vi "MGI RWA Anything to String.vi"(8 "Error In":errorcluster, 9 "Anything":variant, 10 "Read/Write Options":T1={"TS Fmt"="", "Int Fmt"="", "Delimiter"=","}, 11 "Format String (%#_13g)":string="%#_13g") -> (0 "Error Out":errorcluster, 1 "Section":string, 2 "Strings[]":string[](array[string]), 4 "Warnings":string)   [LabVIEW 2023]
doc: "Output a string representation of the specified datatype.\n\nAuthored by Robert C. Mortensen\nsupport@mooregoodideas.com\nwww.mooregoodideas.com\n\nCopyright (c) 2010, Moore Good Ideas, Inc.\n\nAll rights reserved.\n\nRedistribution and use in source and binary forms, with or without modification, are permitted provided that the following conditions are met:\n\n * Redistributions of source code must retain the above copyright notice, this list of conditions and the following disclaimer.\n * Redistributions in binary form must reproduce the above copyright notice, this list of conditions and the following disclaimer in the documentation and/or other materials provided with the distribution.\n * Neither the name of Moore Good Ideas, Inc. nor the names of its contributors may be used to endorse or promote products derived from this software without specific prior written permission.\n\nTHIS SOFTWARE IS PROVIDED BY THE COPYRIGHT HOLDERS AND CONTRIBUTORS \"AS IS\" AND ANY EXPRESS OR IMPLIED WARRANTIES, INCLUDING, BUT NOT LIMITED TO, THE IMPLIED WARRANTIES OF MERCHANTABILITY AND FITNESS FOR A PARTICULAR PURPOSE ARE DISCLAIMED. IN NO EVENT SHALL THE COPYRIGHT OWNER OR CONTRIBUTORS BE LIABLE FOR ANY DIRECT, INDIRECT, INCIDENTAL, SPECIAL, EXEMPLARY, OR CONSEQUENTIAL DAMAGES (INCLUDING, BUT NOT LIMITED TO, PROCUREMENT OF SUBSTITUTE GOODS OR SERVICES; LOSS OF USE, DATA, OR PROFITS; OR BUSINESS INTERRUPTION) HOWEVER CAUSED AND ON ANY THEORY OF LIABILITY, WHETHER IN CONTRACT, STRICT LIABILITY, OR TORT (INCLUDING NEGLIGENCE OR OTHERWISE) ARISING IN ANY WAY OUT OF THE USE OF THIS SOFTWARE, EVEN IF ADVISED OF THE POSSIBILITY OF SUCH DAMAGE."
uses:
  MGI RWA Options Cluster.ctl
  MGI RWA Convertion Direction Enum.ctl
  <vilib>/Utility/Data Type/NI_Data Type.lvlib
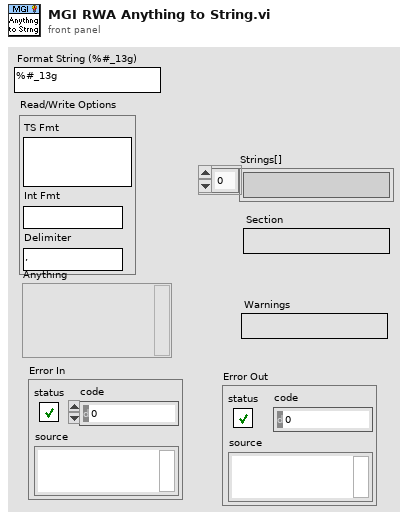
[diagram p1: front panel]
types:
  T1 = typedef "MGI RWA Options Cluster.ctl" = cluster{"TS Fmt":string, "Int Fmt":string, "Delimiter":string}
  T2 = typedef "MGI RWA Convertion Direction Enum.ctl" = enum16{"String->Anything", "Anything->String"}
  T3 = typedef "MGI RWA Tag Lookup Cluster.ctl" = cluster{"StrToSpecifiedText":variant, "Specified Data":variant, "Float Fmt":string, "Major Vers":i32, "Options":T1}
  T4 = typedef "NI_Data Type.lvlib/Data Type.ctl" = enum8{"Invalid Type", "Void", "I8", "I16", "I32", "I64", "U8", "U16", "U32", "U64", "Single Float", "Double Float", "Extended Float", "Single Complex", "Double Complex", "Extended Complex", "Enum U8", "Enum U16", "Enum U32", "Enum U64", "Single Float With Unit", "Double Float With Unit", "Extended Float With Unit", "Single Complex with Unit", "Double Complex with Unit", "Extended Complex with Unit", "Boolean", "String", "Path", "Picture", "Tag", "Array", "Cluster", "Variant", "LV Variant", "Waveform", "Timestamp", "Digital Waveform", "Digital Data", "ExpressData", "Refnum", "External Data", "VI", "Poly VI", "LabVIEW Class Instance", "Fixed Point", "Set Collection", "Map Collection"}
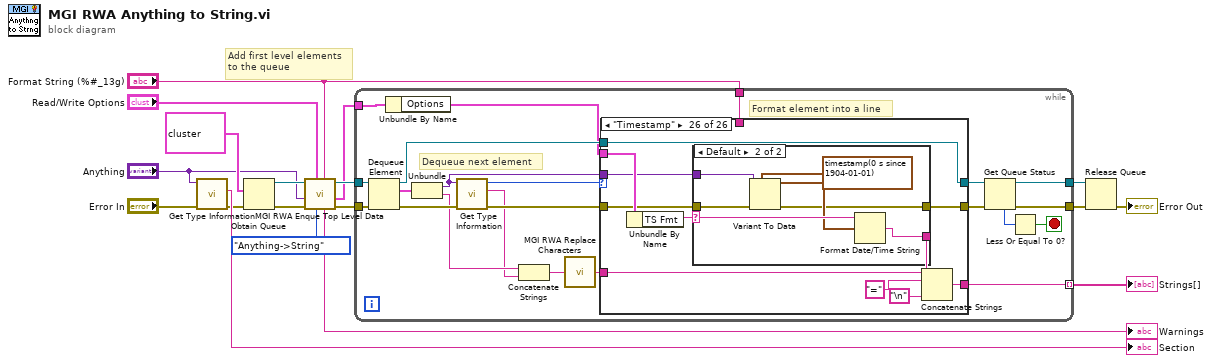
[diagram p0: block diagram]
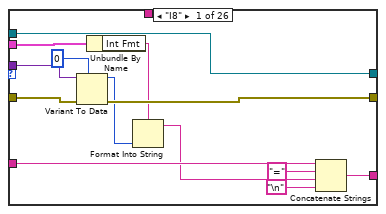
[diagram p2: hidden frame]
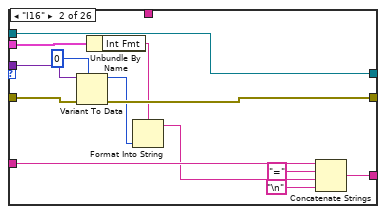
[diagram p3: hidden frame]
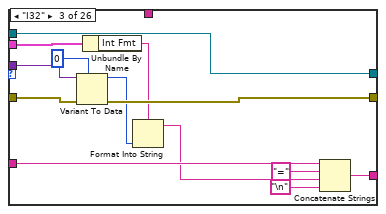
[diagram p4: hidden frame]
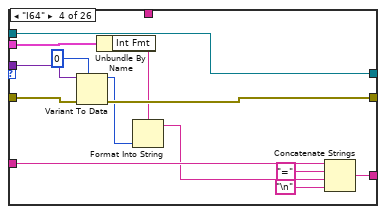
[diagram p5: hidden frame]
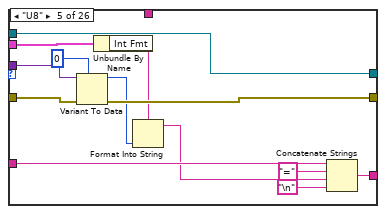
[diagram p6: hidden frame]
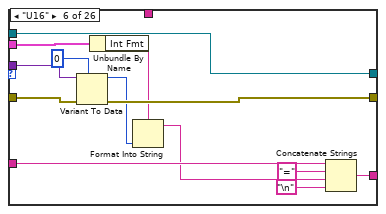
[diagram p7: hidden frame]
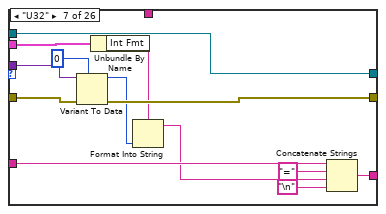
[diagram p8: hidden frame]
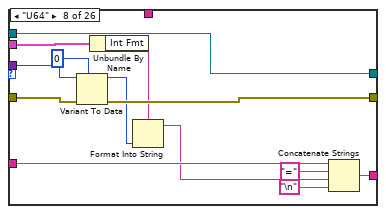
[diagram p9: hidden frame]
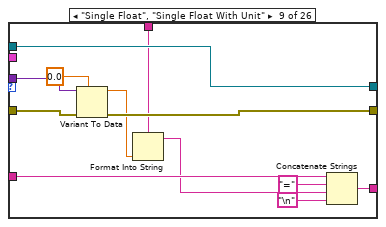
[diagram p10: hidden frame]
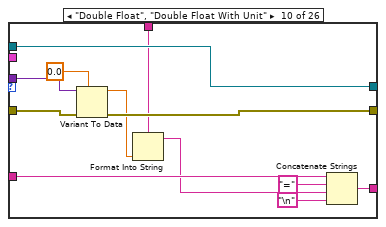
[diagram p11: hidden frame]
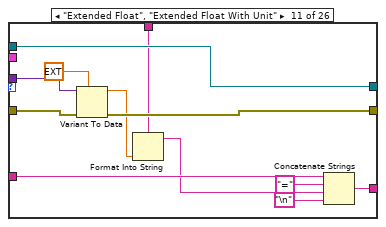
[diagram p12: hidden frame]
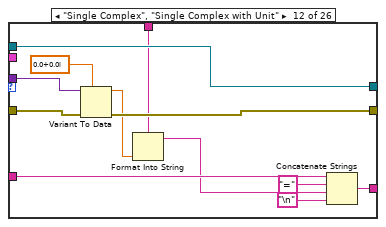
[diagram p13: hidden frame]
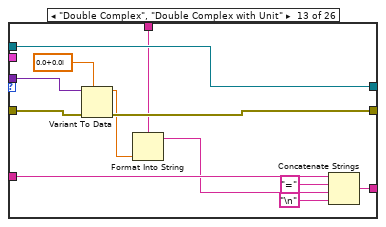
[diagram p14: hidden frame]
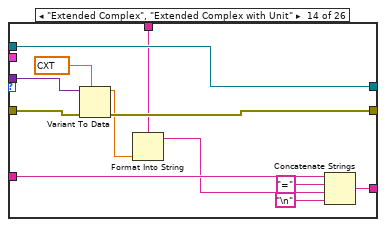
[diagram p15: hidden frame]
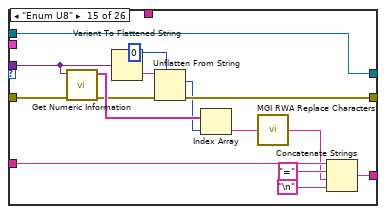
[diagram p16: hidden frame]
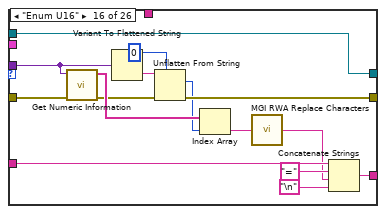
[diagram p17: hidden frame]
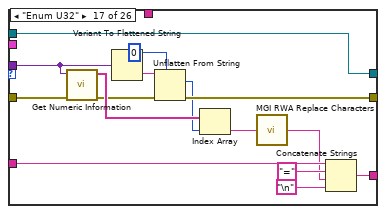
[diagram p18: hidden frame]
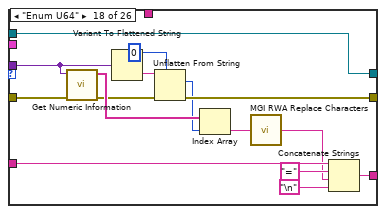
[diagram p19: hidden frame]
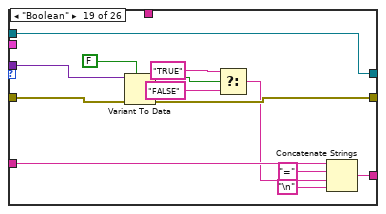
[diagram p20: hidden frame]
diagram:
  # "Add first level elements\nto the queue"
  n1 = call <vilib>:"Get Type Information.vi"("error in (no error)"="Error In", "variant"="Anything") -> ("error out"=w4:errorcluster, "name"=→"Section":string)  [unwired: 5 in, 3 out]
  n2 = Obtain Queue(element data type=cluster{"Variant":variant, "Name":string} {"Variant"=variant, "Name"=""}, error in (no error)=w4) -> (queue out=w10:refnum<queue>, error out=w11:errorcluster)  [unwired: 3 in, 1 out]
  n3 = call "MGI RWA Enque Top Level Data.vi"("Format String (%#_13g)"="Format String (%#_13g)", "Conversion"=MGI_RWA_Convertion_Direction_Enum."Anything->String", "Read/Write Options"="Read/Write Options", "Error In"=w11, "Anything"="Anything", "Data Queue In"=w10) -> ("Error Out"=w6:errorcluster, "Read State"=w2:T3, "Data Queue Our"=w5:refnum<queue>, "Warnings"=→"Warnings":string)  [unwired: 1 in, 1 out]
  n4 = while {
    tunnel: w6 -> [w40]
    tunnel: [w37] -> w12
    tunnel: [w25] -> w18 mode=indexing
    tunnel: w5 -> [w38]
    tunnel: [w34] -> w13
    tunnel: "Format String (%#_13g)" -> [w21]
    tunnel: w2 -> [w20]
    stop <- w35 stop-if-true
    # "Format element into a line"
    # "Dequeue next element"
    n5 = Dequeue Element(queue=w38, error in (no error)=w40) -> (queue out=w31:refnum<queue>, element=w29:cluster{"Variant":variant, "Name":string}, error out=w39:errorcluster)  [unwired: 1 in, 1 out]
    n6 = Unbundle By Name(w20) -> ("Options"=w19:T1)
    n7 = Unbundle(w29) -> ("Variant"=w28:variant, "Name"=w27:string)
    n8 = call <vilib>:"Get Type Information.vi"("error in (no error)"=w39, "variant"=w28) -> ("error out"=w26:errorcluster, "name"=w24:string, "type"=w33:T4)  [unwired: 5 in, 2 out]
    n9 = Concatenate Strings(w27, w24) -> (w23:string)
    n10 = call "MGI RWA Replace Characters.vi"("String In"=w23) -> ("String Out"=w22:string)  [unwired: 1 in]
    n11 = case shown="\"Timestamp\"" w33 {
      selector: w33 -> [_ _ _ _ _ _ _ _ _ _ _ _ _ _ _ _ _ _ _ _ _ _ w330 _ _ _]
      tunnel: [w53 w66 w79 w92 w105 w118 w131 w144 w156 w168 w180 w192 w204 w216 w231 w246 w261 w276 w289 w300 w312 w320 w334 w356 w364 w374] -> w32
      tunnel: w31 -> [w53 w66 w79 w92 w105 w118 w131 w144 w156 w168 w180 w192 w204 w216 w231 w246 w261 w276 w289 w300 w312 w324 w335 w356 w364 w374]
      tunnel: [w49 w62 w75 w88 w101 w114 w127 w140 w152 w164 w176 w188 w200 w212 w225 w240 w255 w270 w288 w292 w311 w321 w336 w355 w363 w367] -> w30
      tunnel: w26 -> [w52 w65 w78 w91 w104 w117 w130 w143 w155 w167 w179 w191 w203 w215 w230 w245 w260 w275 w285 w295 w308 w322 w332 w355 w365 w368]
      tunnel: w22 -> [w46 w58 w71 w84 w97 w110 w123 w136 w148 w160 w172 w183 w195 w207 w219 w234 w249 w264 w278 w296 w303 w316 w326 w345 w359 w373]
      tunnel: w28 -> [w51 w64 w77 w90 w103 w116 w129 w142 w154 w166 w178 w190 w202 w214 w228 w243 w258 w273 w286 w291 w309 w323 w329 w354 w366 w369]
      tunnel: [w45 w59 w72 w85 w98 w111 w124 w137 w149 w161 w173 w184 w196 w208 w220 w235 w250 w265 w279 w297 w304 w317 _ w346 w358 w375] -> w25
      tunnel: w21 -> [_ _ _ _ _ _ _ _ w145 w158 w169 w181 w193 w205 _ _ _ _ _ _ _ w314 _ _ _ _]
      tunnel: w19 -> [w42 w55 w68 w81 w94 w107 w120 w133 _ _ _ _ _ _ _ _ _ _ _ _ _ w313 _ _ _ w371]
      frame "I8" {
        n12 = Variant To Data(error in=w52, type=i8 0, Variant=w51) -> (data=w44:i8, error out=w49:errorcluster)
        n13 = Unbundle By Name(w42) -> ("Int Fmt"=w41:string)
        n14 = Format Into String(format string=w41, w44) -> (resulting string=w43:string)  [unwired: 2 in, 1 out]
        n15 = Concatenate Strings(w46, "=" ("string"), w43, "\n") -> (w45:string)
      }
      frame "I16" {
        n16 = Variant To Data(error in=w65, type=i16 0, Variant=w64) -> (data=w56:i16, error out=w62:errorcluster)
        n17 = Unbundle By Name(w55) -> ("Int Fmt"=w54:string)
        n18 = Format Into String(format string=w54, w56) -> (resulting string=w57:string)  [unwired: 2 in, 1 out]
        n19 = Concatenate Strings(w58, "=" ("string"), w57, "\n") -> (w59:string)
      }
      frame "I32" {
        n20 = Variant To Data(error in=w78, type=0, Variant=w77) -> (data=w70:i32, error out=w75:errorcluster)
        n21 = Unbundle By Name(w68) -> ("Int Fmt"=w67:string)
        n22 = Format Into String(format string=w67, w70) -> (resulting string=w69:string)  [unwired: 2 in, 1 out]
        n23 = Concatenate Strings(w71, "=" ("string"), w69, "\n") -> (w72:string)
      }
      frame "I64" {
        n24 = Variant To Data(error in=w91, type=i64 0, Variant=w90) -> (data=w83:i64, error out=w88:errorcluster)
        n25 = Unbundle By Name(w81) -> ("Int Fmt"=w80:string)
        n26 = Format Into String(format string=w80, w83) -> (resulting string=w82:string)  [unwired: 2 in, 1 out]
        n27 = Concatenate Strings(w84, "=" ("string"), w82, "\n") -> (w85:string)
      }
      frame "U8" {
        n28 = Variant To Data(error in=w104, type=u8 0, Variant=w103) -> (data=w96:u8, error out=w101:errorcluster)
        n29 = Unbundle By Name(w94) -> ("Int Fmt"=w93:string)
        n30 = Format Into String(format string=w93, w96) -> (resulting string=w95:string)  [unwired: 2 in, 1 out]
        n31 = Concatenate Strings(w97, "=" ("string"), w95, "\n") -> (w98:string)
      }
      frame "U16" {
        n32 = Variant To Data(error in=w117, type=u16 0, Variant=w116) -> (data=w109:u16, error out=w114:errorcluster)
        n33 = Unbundle By Name(w107) -> ("Int Fmt"=w106:string)
        n34 = Format Into String(format string=w106, w109) -> (resulting string=w108:string)  [unwired: 2 in, 1 out]
        n35 = Concatenate Strings(w110, "=" ("string"), w108, "\n") -> (w111:string)
      }
      frame "U32" {
        n36 = Variant To Data(error in=w130, type=u32 0, Variant=w129) -> (data=w122:u32, error out=w127:errorcluster)
        n37 = Unbundle By Name(w120) -> ("Int Fmt"=w119:string)
        n38 = Format Into String(format string=w119, w122) -> (resulting string=w121:string)  [unwired: 2 in, 1 out]
        n39 = Concatenate Strings(w123, "=" ("string"), w121, "\n") -> (w124:string)
      }
      frame "U64" {
        n40 = Variant To Data(error in=w143, type=u64 0, Variant=w142) -> (data=w135:u64, error out=w140:errorcluster)
        n41 = Unbundle By Name(w133) -> ("Int Fmt"=w132:string)
        n42 = Format Into String(format string=w132, w135) -> (resulting string=w134:string)  [unwired: 2 in, 1 out]
        n43 = Concatenate Strings(w136, "=" ("string"), w134, "\n") -> (w137:string)
      }
      frame "Single Float", "Single Float With Unit" {
        n44 = Variant To Data(error in=w155, type=sgl 0.0, Variant=w154) -> (data=w147:sgl, error out=w152:errorcluster)
        n45 = Format Into String(format string=w145, w147) -> (resulting string=w146:string)  [unwired: 2 in, 1 out]
        n46 = Concatenate Strings(w148, "=" ("string"), w146, "\n") -> (w149:string)
      }
      frame "Double Float", "Double Float With Unit" {
        n47 = Variant To Data(error in=w167, type=0.0, Variant=w166) -> (data=w159:dbl, error out=w164:errorcluster)
        n48 = Format Into String(format string=w158, w159) -> (resulting string=w157:string)  [unwired: 2 in, 1 out]
        n49 = Concatenate Strings(w160, "=" ("string"), w157, "\n") -> (w161:string)
      }
      frame "Extended Float", "Extended Float With Unit" {
        n50 = Variant To Data(error in=w179, type=ext 0.0, Variant=w178) -> (data=w171:ext, error out=w176:errorcluster)
        n51 = Format Into String(format string=w169, w171) -> (resulting string=w170:string)  [unwired: 2 in, 1 out]
        n52 = Concatenate Strings(w172, "=" ("string"), w170, "\n") -> (w173:string)
      }
      frame "Single Complex", "Single Complex with Unit" {
        n53 = Variant To Data(error in=w191, type=csg 0.0+0.0i, Variant=w190) -> (data=w187:csg, error out=w188:errorcluster)
        n54 = Format Into String(format string=w181, w187) -> (resulting string=w182:string)  [unwired: 2 in, 1 out]
        n55 = Concatenate Strings(w183, "=" ("string"), w182, "\n") -> (w184:string)
      }
      frame "Double Complex", "Double Complex with Unit" {
        n56 = Variant To Data(error in=w203, type=cdb 0.0+0.0i, Variant=w202) -> (data=w199:cdb, error out=w200:errorcluster)
        n57 = Format Into String(format string=w193, w199) -> (resulting string=w194:string)  [unwired: 2 in, 1 out]
        n58 = Concatenate Strings(w195, "=" ("string"), w194, "\n") -> (w196:string)
      }
      frame "Extended Complex", "Extended Complex with Unit" {
        n59 = Variant To Data(error in=w215, type=cxt 0.0+0.0i, Variant=w214) -> (data=w211:cxt, error out=w212:errorcluster)
        n60 = Format Into String(format string=w205, w211) -> (resulting string=w206:string)  [unwired: 2 in, 1 out]
        n61 = Concatenate Strings(w207, "=" ("string"), w206, "\n") -> (w208:string)
      }
      frame "Enum U8" {
        n62 = call <vilib>:"Get Numeric Information.vi"("error in (no error)"=w230, "variant"=w228) -> ("error out"=w226:errorcluster, "enum names"=w229:string[])  [unwired: 6 in, 2 out]
        n63 = Variant To Flattened String(Variant=w228) -> (data string=w227:string)  [unwired: 1 out]
        n64 = Unflatten From String(type=u8 0, binary string=w227, error in (no error)=w226) -> (value=w224:u8, error out=w225:errorcluster)  [unwired: 2 in, 1 out]
        n65 = Index Array(array=w229, index=w224) -> (element=w218:string)
        n66 = call "MGI RWA Replace Characters.vi"("String In"=w218) -> ("String Out"=w217:string)  [unwired: 1 in]
        n67 = Concatenate Strings(w219, "=" ("string"), w217, "\n") -> (w220:string)
      }
      frame "Enum U16" {
        n68 = call <vilib>:"Get Numeric Information.vi"("error in (no error)"=w245, "variant"=w243) -> ("error out"=w241:errorcluster, "enum names"=w244:string[])  [unwired: 6 in, 2 out]
        n69 = Variant To Flattened String(Variant=w243) -> (data string=w242:string)  [unwired: 1 out]
        n70 = Unflatten From String(type=u16 0, binary string=w242, error in (no error)=w241) -> (value=w239:u16, error out=w240:errorcluster)  [unwired: 2 in, 1 out]
        n71 = Index Array(array=w244, index=w239) -> (element=w233:string)
        n72 = call "MGI RWA Replace Characters.vi"("String In"=w233) -> ("String Out"=w232:string)  [unwired: 1 in]
        n73 = Concatenate Strings(w234, "=" ("string"), w232, "\n") -> (w235:string)
      }
      frame "Enum U32" {
        n74 = call <vilib>:"Get Numeric Information.vi"("error in (no error)"=w260, "variant"=w258) -> ("error out"=w256:errorcluster, "enum names"=w259:string[])  [unwired: 6 in, 2 out]
        n75 = Variant To Flattened String(Variant=w258) -> (data string=w257:string)  [unwired: 1 out]
        n76 = Unflatten From String(type=u32 0, binary string=w257, error in (no error)=w256) -> (value=w254:u32, error out=w255:errorcluster)  [unwired: 2 in, 1 out]
        n77 = Index Array(array=w259, index=w254) -> (element=w248:string)
        n78 = call "MGI RWA Replace Characters.vi"("String In"=w248) -> ("String Out"=w247:string)  [unwired: 1 in]
        n79 = Concatenate Strings(w249, "=" ("string"), w247, "\n") -> (w250:string)
      }
      frame "Enum U64" {
        n80 = call <vilib>:"Get Numeric Information.vi"("error in (no error)"=w275, "variant"=w273) -> ("error out"=w271:errorcluster, "enum names"=w274:string[])  [unwired: 6 in, 2 out]
        n81 = Variant To Flattened String(Variant=w273) -> (data string=w272:string)  [unwired: 1 out]
        n82 = Unflatten From String(type=u64 0, binary string=w272, error in (no error)=w271) -> (value=w269:u64, error out=w270:errorcluster)  [unwired: 2 in, 1 out]
        n83 = Index Array(array=w274, index=w269) -> (element=w263:string)
        n84 = call "MGI RWA Replace Characters.vi"("String In"=w263) -> ("String Out"=w262:string)  [unwired: 1 in]
        n85 = Concatenate Strings(w264, "=" ("string"), w262, "\n") -> (w265:string)
      }
      frame "Boolean" {
        n86 = Variant To Data(error in=w285, type=FALSE, Variant=w286) -> (data=w284:bool, error out=w288:errorcluster)
        n87 = Select(t="TRUE", s=w284, f="FALSE") -> (s? t:f=w277:string)
        n88 = Concatenate Strings(w278, "=" ("string"), w277, "\n") -> (w279:string)
      }
      frame "String" {
        n89 = Variant To Data(error in=w295, type="", Variant=w291) -> (data=w294:string, error out=w292:errorcluster)
        n90 = call "MGI RWA Replace Characters.vi"("String In"=w294) -> ("String Out"=w293:string)  [unwired: 1 in]
        n91 = Concatenate Strings(w296, "=" ("string"), w293, "\n") -> (w297:string)
      }
      frame "Path" {
        n92 = Variant To Data(error in=w308, type=path "", Variant=w309) -> (data=w307:path, error out=w311:errorcluster)
        n93 = Path To String(path=w307) -> (string=w302:string)
        n94 = call "MGI RWA Replace Characters.vi"("String In"=w302) -> ("String Out"=w301:string)  [unwired: 1 in]
        n95 = Concatenate Strings(w303, "=" ("string"), w301, "\n") -> (w304:string)
      }
      frame "Array" {
        n96 = call "MGI RWA Process Array Elements.vi"("Read/Write Options"=w313, "Format String (%#0.15f)"=w314, "Error In"=w322, "Name In"=w316, "Array Variant"=w323, "Queue In"=w324) -> ("Error Out"=w321:errorcluster, "Data Out"=w315:string, "Queue Out"=w320:refnum<queue>)  [unwired: 3 in]
        n97 = Concatenate Strings(w316, "=" ("string"), w315, "\n") -> (w317:string)
      }
      frame "Cluster" {
        # "Enqueue cluster elements"
        n98 = call "MGI Get Cluster Elements.vi"("Error In"=w332, "Cluster"=w329, "Type Enum (Cluster)"=w330) -> ("Error Out"=w331:errorcluster, "Cluster Elements"=w328:variant[])  [unwired: 7 in]
        n99 = Concatenate Strings(w326, "." ("string")) -> (w325:string)
        n100 = Reverse 1D Array(array=w328) -> (reversed array=w333:variant[])
        n101 = for {
          tunnel: w335 -> [w343]
          tunnel: w331 -> [w342]
          tunnel: [w341] -> w336
          tunnel: [w340] -> w334
          tunnel: w333 -> [w338] mode=indexing
          tunnel: w325 -> [w337]
          n102 = Bundle("Variant"=w338, w337) -> (w339:cluster{"Variant":variant, string})  [unwired: 1 in]
          n103 = Enqueue Element At Opposite End(queue=w343, element=w339, error in (no error)=w342) -> (queue out=w340:refnum<queue>, error out=w341:errorcluster)  [unwired: 1 in, 1 out]
        }
      }
      frame Default {
        n104 = Variant To Flattened String(Variant=w354) -> (data string=w349:string)  [unwired: 1 out]
        n105 = String To Byte Array(string=w349) -> (unsigned byte array=w353:u8[])
        n106 = Number To Hexadecimal String(1:i16 2 ("width (-)"), 2:w353) -> (0:w352:string[])
        n107 = Concatenate Strings("0x", w352) -> (w344:string)
        n108 = Concatenate Strings(w345, "=" ("string"), w344, "\n") -> (w346:string)
      }
      frame "Tag", "Refnum" {
        n109 = call "MGI RWA Handle Tag or Refnum.vi"("Conversion"=MGI_RWA_Convertion_Direction_Enum."Anything->String", "Error In"=w365, "Anything"=w366) -> ("Error Out"=w363:errorcluster, "String"=w360:string)  [unwired: 7 in]
        n110 = Concatenate Strings(w359, "=" ("string"), w360, "\n") -> (w358:string)
      }
      frame "Timestamp" {
        n111 = Unbundle By Name(w371) -> ("TS Fmt"=w370:string)
        n112 = case shown="Default" w370 {
          selector: w370 -> [_ w391]
          tunnel: [w381 w392] -> w372
          tunnel: w369 -> [w380 w389]
          tunnel: w368 -> [w378 w388]
          tunnel: [w378 w386] -> w367
          frame "" {
            n113 = Variant To Flattened String(Variant=w380) -> (data string=w379:string)  [unwired: 1 out]
            n114 = String To Byte Array(string=w379) -> (unsigned byte array=w384:u8[])
            n115 = Number To Hexadecimal String(1:i16 2 ("width (-)"), 2:w384) -> (0:w383:string[])
            n116 = Concatenate Strings("0x", w383) -> (w381:string)
          }
          frame Default {
            n117 = Variant To Data(error in=w388, type=timestamp(0 s since 1904-01-01), Variant=w389) -> (data=w387:timestamp, error out=w386:errorcluster)
            n118 = Format Date/Time String(time format string (%c)=w391, seconds (now)=w387) -> (date/time string=w392:string)  [unwired: 1 in]
          }
        }
        n119 = Concatenate Strings(w373, "=" ("string"), w372, "\n") -> (w375:string)
      }
    }
    n120 = Get Queue Status(queue=w32, error in (no error)=w30) -> (queue out=w34:refnum<queue>, error out=w37:errorcluster, # elements in queue=w36:i32)  [unwired: 1 in, 5 out]
    n121 = Less Or Equal To 0?(x=w36) -> (x <= 0?=w35:bool)
  }
  "Strings[]" <- w18
  n122 = Release Queue(queue=w13, error in (no error)=w12) -> (error out=→"Error Out":errorcluster)  [unwired: 1 in, 2 out]
